vi "Read All Data.vi"() -> ()   [LabVIEW 2012]
doc: "This example returns data from the database you choose using the Connection Information, Username, and Password.\n\nA list of the database tables appears in the Table Names menu ring. You can then press the Get Data button to return all the data from the selected table into the Table Data indicator. The numbers of rows and columns in that table are also returned in the respective indicators. You press the Stop button when you are finished with the example. \n\nThis example was written to solve a unique problem associated with reading very large recordsets where the performance becomes slow from the use of a large amount of computer resources. SubVIs named DB Tools Select All Data and DB Tools Fetch Table Data have been optimized to use the least number of resources and thus provide the best performance when reading large recordsets."
uses:
  NI_Database_API_64.lvlib
  Connection.llb/DB Tools Open Connec (String).vi
panel:
  in  "Password":string
  in  "Username":string
  in  "Connection Information":string="LabVIEW"
  out "Columns":i32
  out "Rows":i32
  in  "Get Value":bool
  in  "stop":bool
  in  "Table Names":u16(ring) items=["fetchdata", "fetchempty", "inserttable", "logging", "parameterized", "sixtypes"]
  out "Table Data":string[][](table)
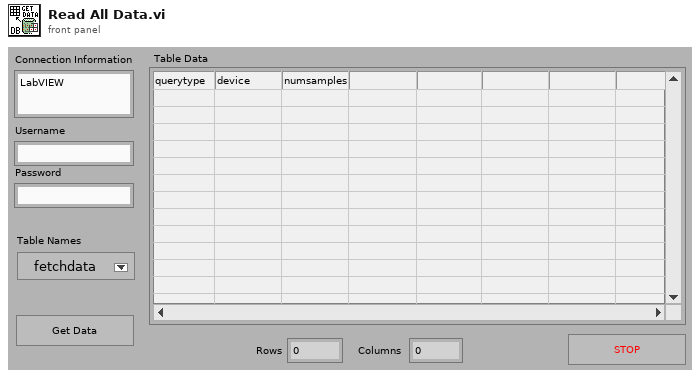
[diagram p1: front panel]
types:
  T1 = typedef "NI_Database_API_64.lvlib/Conn ObjectReference.ctl" = refnum<k1>
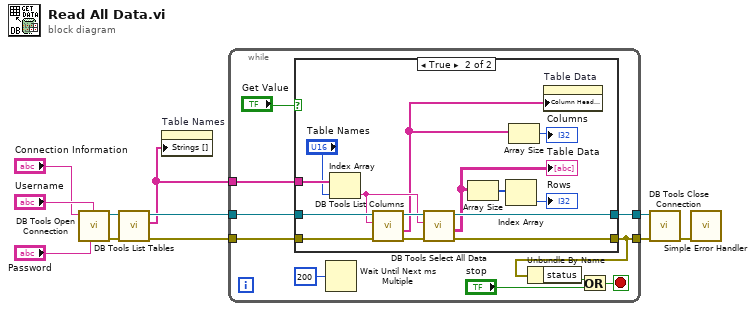
[diagram p0: block diagram]
diagram:
  n1 = call-poly "DB Tools Open Connection.vi"("password"="Password", "userID"="Username", "connection information"="Connection Information") -> ("error out"=w7:errorcluster, "connection reference"=w8:T1)  [unwired: 5 in]
  n2 = call "DB Tools List Tables.vi"("error in (no error)"=w7, "connection reference"=w8) -> ("error out"=w6:errorcluster, "tables"=w4:string[], "connection reference out"=w5:T1)  [unwired: 3 in]
  n3 = property on="Table Names" class="Ring (strict)"("Strings []"=w4) -> ()  [unwired: 2 in, 2 out]
  n4 = while {
    tunnel: [w21] -> w11
    tunnel: [w12] -> w9
    tunnel: w6 -> [w20]
    tunnel: w5 -> [w19]
    tunnel: w4 -> [w18]
    stop <- w15 stop-if-true
    n5 = case shown="True" "Get Value" {
      tunnel: [w22 w37] -> w21
      tunnel: [w23 w24] -> w12
      tunnel: w20 -> [w23 w33]
      tunnel: w19 -> [w22 w32]
      tunnel: w18 -> [_ w31]
      frame False {
      }
      frame True {
        n6 = Index Array(array=w31, index="Table Names") -> (element=w30:string)
        n7 = call "DB Tools List Columns.vi"("error in (no error)"=w33, "table"=w30, "connection reference"=w32) -> ("error out"=w35:errorcluster, "columns"=w26:string[], "connection reference out"=w36:T1)  [unwired: 1 in, 1 out]
        n8 = call "DB Tools Select All Data.vi"("error in (no error)"=w35, "table"=w30, "connection reference"=w36) -> ("error out"=w24:errorcluster, "data"=w34:string[][], "connection reference out"=w37:T1)  [unwired: 3 in]
        "Table Data" <- w34
        n9 = Array Size(array=w34) -> (size(s)=w28:i32[])
        n10 = Index Array(array=w28) -> (element=→"Rows":i32)  [unwired: 1 in]
        n11 = Array Size(array=w26) -> (size(s)=→"Columns":i32)
        n12 = property on="Table Data" class="Tbl (strict)"("Column Header Strings[]"=w26) -> ()  [unwired: 2 in, 2 out]
      }
    }
    n13 = Wait Until Next ms Multiple(millisecond multiple=u32 200) -> ()  [unwired: 1 out]
    n14 = Unbundle By Name(w12) -> ("status"=w13:bool)
    n15 = Or(x=w13, y="stop") -> (x .or. y?=w15:bool)
  }
  n16 = call "DB Tools Close Connection.vi"("error in (no error)"=w9, "connection reference"=w11) -> ("error out"=w10:errorcluster)  [unwired: 5 in]
  n17 = call <vilib>:"Simple Error Handler.vi"("error in (no error)"=w10) -> ()  [unwired: 4 in, 5 out]
